vi "Update Scrollbar.vi"(4 "Area Height":u32, 5 "Display State In":T4={"Current Channels Info"=[], "Help Prefix"="", "Max Display Size"=8, "Max Size"=8, "Show Buttons"=TRUE, "Data Valid"=refnum, "Show Range"=FALSE, "Range Items"=[], "Range Index"=[]} caption="State", 7 "Channels In":T1, 8 "error in (no error)":errorcluster, 9 "Current Index":i32, 11 "Scrollbar Reference":refnum<vi>) -> (0 "error out":errorcluster)   [LabVIEW 2021, in "myRIO Channel List.xctl"]
uses:
  <vilib>/myRIO/Common/Express VI Framework/xctls/myRIO Channel List/myRIO Channel List.xctl
  <vilib>/myRIO/Common/Express VI Framework/xctls/myRIO Channel List/State.ctl
  <vilib>/myRIO/Common/Profile Manager Framework/typedefs/Channel Info.ctl
  <vilib>/myRIO/Common/Express VI Framework/typedefs/Data Validate Ref.ctl
  <vilib>/myRIO/Common/Express VI Framework/xctls/myRIO Channel List/Data.ctl
  <vilib>/myRIO/Common/Express VI Framework/xctls/myRIO Channel List/typedefs/Channel Data.ctl
  <vilib>/myRIO/Common/Express VI Framework/xctls/myRIO Channel List/typedefs/Remove Channel.ctl
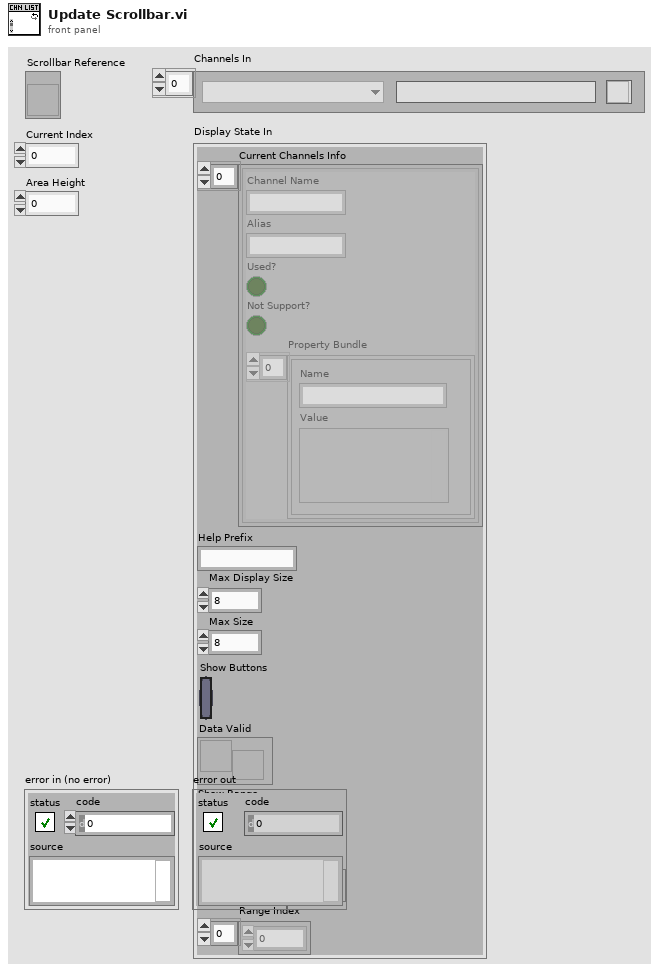
[diagram p1: front panel]
types:
  T1 = typedef "myRIO Channel List.xctl/Data.ctl" = T2[]
  T2 = typedef "myRIO Channel List.xctl/Channel Data.ctl" = cluster{"Channel Name":u16, "Channel Alias":string, "Remove Channel":T3, "Index":i32}
  T3 = typedef "myRIO Channel List.xctl/Remove Channel.ctl" = bool
  T4 = typedef "myRIO Channel List.xctl/State.ctl" = cluster{"Current Channels Info":T5[], "Help Prefix":string, "Max Display Size":i32, "Max Size":i32, "Show Buttons":bool, "Data Valid":T6, "Show Range":bool, "Range Items":string[], "Range Index":i32[]}
  T5 = typedef "Channel Info.ctl" = cluster{"Channel Name":string, "Alias":string, "Used?":bool, "Not Support?":bool, "Property Bundle":cluster{"Name":string, "Value":variant}[]}
  T6 = typedef "Data Validate Ref.ctl" = refnum<user-event>
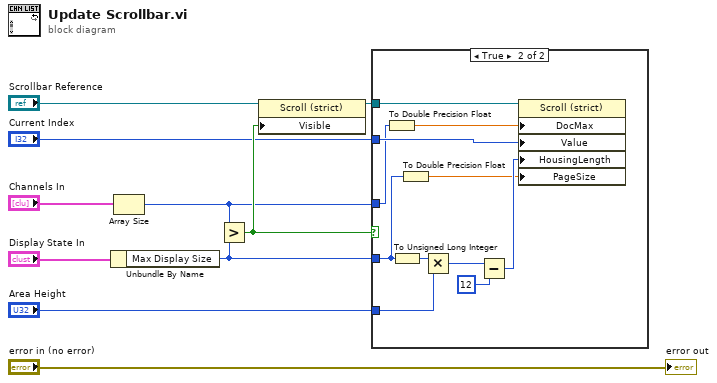
[diagram p0: block diagram]
diagram:
  n1 = Unbundle By Name("Display State In") -> ("Max Display Size"=w4:i32)
  n2 = Array Size(array="Channels In") -> (size(s)=w5:i32)
  n3 = Greater?(x=w5, y=w4) -> (0:w7:bool)
  n4 = property class="Scroll (strict)"(reference="Scrollbar Reference", "Visible"=w7) -> (reference out=w6:refnum<vi>)  [unwired: 1 in, 1 out]
  n5 = case shown="True" w7 {
    tunnel: w6 -> [_ w21]
    tunnel: w5 -> [_ w13]
    tunnel: w4 -> [_ w12]
    tunnel: "Current Index" -> [_ w14]
    tunnel: "Area Height" -> [_ w18]
    frame False {
    }
    frame True {
      n6 = To Double Precision Float(number=w13) -> (double precision float=w15:dbl)
      n7 = To Unsigned Long Integer(number=w12) -> (unsigned 32bit integer=w16:u32)
      n8 = To Double Precision Float(number=w12) -> (double precision float=w11:dbl)
      n9 = Multiply(x=w16, y=w18) -> (x*y=w20:u32)
      n10 = Subtract(x=w20, y=u32 12) -> (x-y=w17:u32)
      n11 = property class="Scroll (strict)"(reference=w21, "DocMax"=w15, "Value"=w14, "HousingLength"=w17, "PageSize"=w11) -> ()  [unwired: 1 in, 2 out]
    }
  }
  "error out" <- "error in (no error)"
